vi "03 WriteOff.vi"(8 "error in (no error)":errorcluster caption="错误输入（无错误）", 11 "TCPServerClass 输入":refnum<class "TCPServerClass.lvclass">) -> (0 "error out":errorcluster caption="错误输出", 3 "TCPServerClass 输出":refnum<class "TCPServerClass.lvclass">)   [LabVIEW 2019, in "TCPServerClass.lvclass"]
uses:
  TCPServerClass.lvclass
  TCPServerClass.lvclass/TCPServerClass.ctl
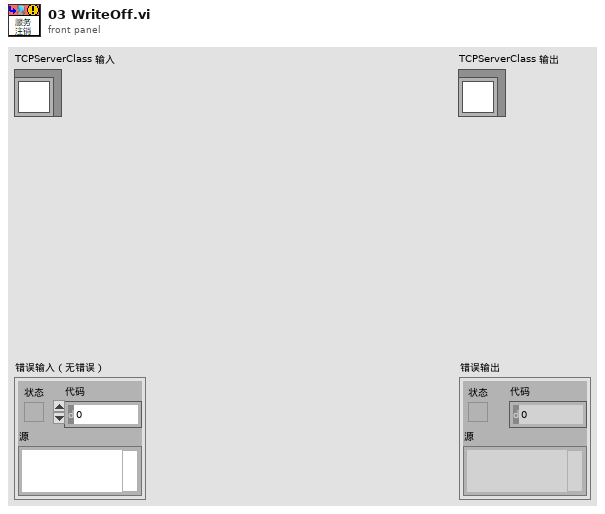
[diagram p1: front panel]
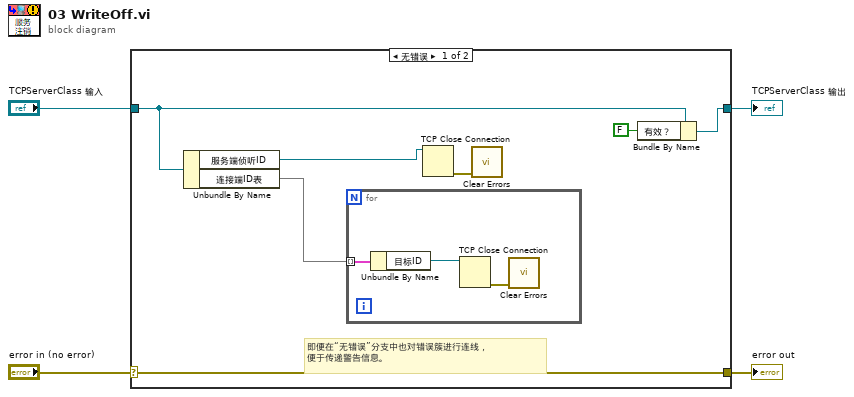
[diagram p0: block diagram]
diagram:
  n1 = case shown="无错误" "error in (no error)" {
    selector: "error in (no error)" -> [w11 w16]
    tunnel: [w11 w16] -> w3
    tunnel: [w5 w15] -> w1
    tunnel: "TCPServerClass 输入" -> [w7 w15]
    frame No Error {
      # "即便在“无错误”分支中也对错误簇进行连线，\n便于传递警告信息。"
      n2 = Unbundle By Name(w7) -> ("服务端侦听ID"=w10:refnum<k5>, "连接端ID表"=w8:map{string, refnum<k5>})
      n3 = for {
        tunnel: w8 -> [w14] mode=indexing
        n4 = Unbundle By Name(w14) -> ("目标ID"=w12:refnum<k5>)
        n5 = TCP Close Connection(connection ID=w12) -> (error out=w13:errorcluster)  [unwired: 2 in, 1 out]
        n6 = call <vilib>:"Clear Errors.vi"("error in (no error)"=w13) -> ()  [unwired: 5 in, 2 out]
      }
      n7 = TCP Close Connection(connection ID=w10) -> (error out=w9:errorcluster)  [unwired: 2 in, 1 out]
      n8 = call <vilib>:"Clear Errors.vi"("error in (no error)"=w9) -> ()  [unwired: 5 in, 2 out]
      n9 = Bundle By Name(cluster=w7, "有效？"=FALSE) -> (w5:refnum<class "TCPServerClass.lvclass">)
    }
    frame Error {
    }
  }
  "error out" <- w3
  "TCPServerClass 输出" <- w1
